vi "Cycle History Read.vi"(0 "GEA2 Reference In":refnum<k24>, 5 "Standalone?":bool, 6 "Cycle History Buffer Selection":T1, 11 "Error In":errorcluster) -> (4 "GEA2 Reference Out":refnum<k24>, 8 "output cluster":T2, 15 "Error Out":errorcluster)   [LabVIEW 2016, in "TL27.lvlib"]
uses:
  Projects/TL27.lvlib
  Q:/Common/DLLs/GEA3/GeaCommunication.dll
  Common/DLLs/GEA3/GeaCommunication.dll
  type defs/Cycle_Diag_Teststand.ctl
  type defs/Cycle History Buffer Selector.ctl
  Common/LabVIEW GEA2 Toolkit/LabVIEW_GEA2_Toolkit.lvlibp/type defs/Source_Destination.ctl
  Common/LabVIEW GEA2 Toolkit/LabVIEW_GEA2_Toolkit.lvlibp/type defs/ERD Read Data In.ctl
  Common/LabVIEW GEA2 Toolkit/LabVIEW_GEA2_Toolkit.lvlibp/type defs/Data Type.ctl
  Common/LabVIEW GEA2 Toolkit/LabVIEW_GEA2_Toolkit.lvlibp
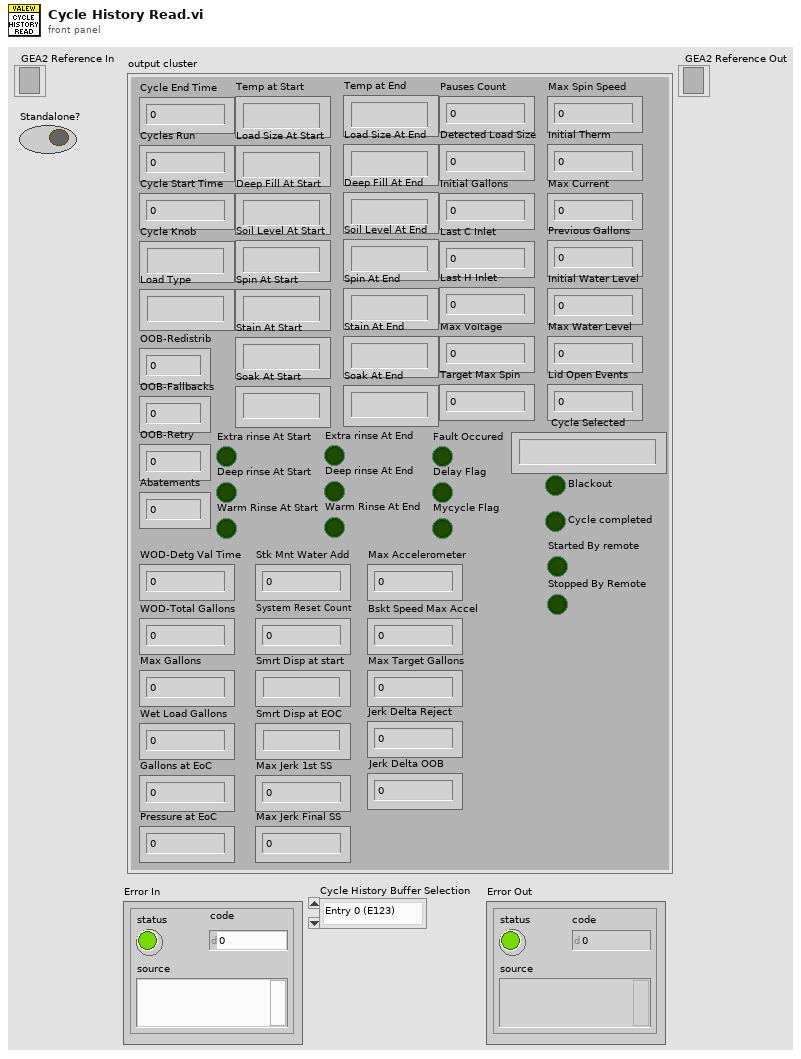
[diagram p1: front panel]
types:
  T1 = typedef "TL27.lvlib/Cycle History Buffer Selector.ctl" = enum16{"Entry 0 (E123)", "Entry 1 (E124)", "Entry 2 (E125)", "Entry 3 (E126)", "Entry 4 (E127)", "Entry 5 (E128)", "Entry 6 (E129)", "Entry 7 (E12A)", "Entry 8 (E12B)", "Entry 9 (E12C)"}
  T2 = typedef "TL27.lvlib/Cycle_Diag_Teststand.ctl" = cluster{"Cycle End Time":u32, "Cycles Run":u32, "Cycle Start Time":u32, "Cycle Knob":string, "Load Type":string, "OOB-Redistrib":u8, "OOB-Fallbacks":u8, "OOB-Retry":u8, "Temp at Start":string, "Load Size At Start":string, "Deep Fill At Start":string, "Soil Level At Start":string, "Spin At Start":string, "Extra rinse At Start":bool, "Deep rinse At Start":bool, "Stain At Start":string, "Soak At Start":string, "Warm Rinse At Start":bool, "Temp at End":string, "Load Size At End":string, "Deep Fill At End":string, "Soil Level At End":string, "Spin At End":string, "Extra rinse At End":bool, "Deep rinse At End":bool, "Stain At End":string, "Soak At End":string, "Warm Rinse At End":bool, "Pauses Count":u8, "Fault Occured":bool, "Delay Flag":bool, "Mycycle Flag":bool, "Blackout":bool, "Cycle completed":bool, "Detected Load Size":dbl, "Initial Gallons":dbl, "Last C Inlet ":dbl, "Max Voltage":dbl, "Target Max Spin":u16, "Max Spin Speed":u16, "Initial Therm":dbl, "Max Current":dbl, "Previous Gallons":dbl, "Initial Water Level":dbl, "Max Water Level":dbl, "Abatements ":u8, "Lid Open Events":u8, "Cycle Selected":string, "Last H Inlet ":dbl, "WOD-Detg Val Time":u8, "WOD-Total Gallons":u16, "Max Gallons":u16, "Wet Load Gallons":u16, "Gallons at EoC":u16, "Pressure at EoC":u32, "Stk Mnt Water Add":u8, "Started By remote":bool, "Stopped By Remote":bool, "System Reset Count":u8, "Smrt Disp at start":string, "Smrt Disp at EOC":string, "Max Jerk 1st SS":i32, "Max Jerk Final SS":i32, "Max Accelerometer":i16, "Bskt Speed Max Accel":u16, "Max Target Gallons":u16, "Jerk Delta Reject":u8, "Jerk Delta OOB ":u8}
  T3 = typedef "LabVIEW_GEA2_Toolkit.lvlibp/Source_Destination.ctl" = cluster{"Source":u8, "Destination":u8}
  T4 = typedef "LabVIEW_GEA2_Toolkit.lvlibp/ERD Read Data In.ctl" = cluster{"ERD Number":u16, "Data Type":T5}
  T5 = typedef "LabVIEW_GEA2_Toolkit.lvlibp/Data Type.ctl" = enum16{"string", "boolean", "uint8_t", "uint16_t", "uint32_t", "uint64_t", "int8_t", "int16_t", "int32_t", "int64_t"}
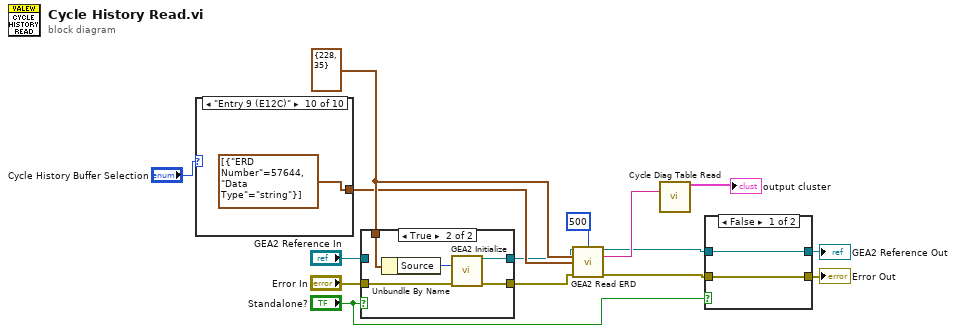
[diagram p0: block diagram]
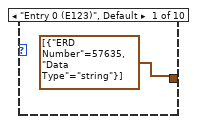
[diagram p2: hidden frame]
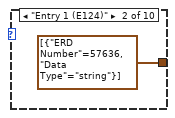
[diagram p3: hidden frame]
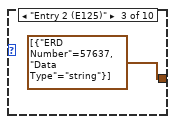
[diagram p4: hidden frame]
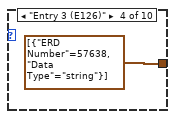
[diagram p5: hidden frame]
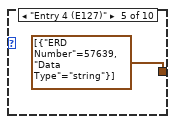
[diagram p6: hidden frame]
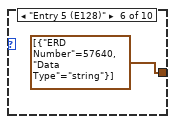
[diagram p7: hidden frame]
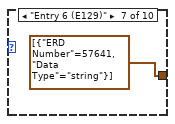
[diagram p8: hidden frame]
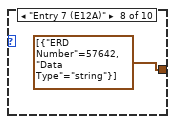
[diagram p9: hidden frame]
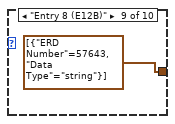
[diagram p10: hidden frame]
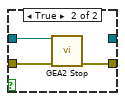
[diagram p11: hidden frame]
diagram:
  w9 = T3 {"Source"=228, "Destination"=35} ("GEA Inputs")
  n1 = case shown="\"Entry 9 (E12C)\"" "Cycle History Buffer Selection" {
    tunnel: [T4[] [{"ERD Number"=57635, "Data Type"=enum."string"}] ("Read ERD List") T4[] [{"ERD Number"=57636, "Data Type"=enum."string"}] ("Read ERD List") T4[] [{"ERD Number"=57637, "Data Type"=enum."string"}] ("Read ERD List") T4[] [{"ERD Number"=57638, "Data Type"=enum."string"}] ("Read ERD List") T4[] [{"ERD Number"=57639, "Data Type"=enum."string"}] ("Read ERD List") T4[] [{"ERD Number"=57640, "Data Type"=enum."string"}] ("Read ERD List") T4[] [{"ERD Number"=57641, "Data Type"=enum."string"}] ("Read ERD List") T4[] [{"ERD Number"=57642, "Data Type"=enum."string"}] ("Read ERD List") T4[] [{"ERD Number"=57643, "Data Type"=enum."string"}] ("Read ERD List") T4[] [{"ERD Number"=57644, "Data Type"=enum."string"}] ("Read ERD List")] -> w7
    frame "Entry 0 (E123)", Default {
    }
    frame "Entry 1 (E124)" {
    }
    frame "Entry 2 (E125)" {
    }
    frame "Entry 3 (E126)" {
    }
    frame "Entry 4 (E127)" {
    }
    frame "Entry 5 (E128)" {
    }
    frame "Entry 6 (E129)" {
    }
    frame "Entry 7 (E12A)" {
    }
    frame "Entry 8 (E12B)" {
    }
    frame "Entry 9 (E12C)" {
    }
  }
  n2 = case shown="True" "Standalone?" {
    tunnel: "Error In" -> [w26 w32]
    tunnel: [w26 w31] -> w10
    tunnel: "GEA2 Reference In" -> [w27 _]
    tunnel: [w27 w30] -> w6
    tunnel: w9 -> [_ w28]
    frame False {
    }
    frame True {
      n3 = Unbundle By Name(w28) -> ("Source"=w29:u8)
      n4 = call "GEA2 Initialize.vi"("Source Address"=w29, "error in"=w32) -> ("GEA2 Reference Out"=w30:refnum<k24>, "error out"=w31:errorcluster)  [unwired: 11 in, 1 out]
    }
  }
  n5 = call "GEA2 Read ERD.vi"("GEA2 Reference In"=w6, "Read Timeout (ms)"=u32 500, "GEA Inputs"=w9, "Read ERD List"=w7, "Error In"=w10) -> ("GEA2 Reference Out"=w4:refnum<k24>, "Raw Data Out"=w5:string, "Error Out"=w3:errorcluster)  [unwired: 7 in, 1 out]
  n6 = call "Cycle Diag Table Read.vi"("Raw Data In"=w5) -> ("output cluster"=→"output cluster":T2)  [unwired: 14 in]
  n7 = case shown="False" "Standalone?" {
    tunnel: [w33 w37] -> w13
    tunnel: w4 -> [w34 w36]
    tunnel: [w34 _] -> w12
    tunnel: w3 -> [w33 w35]
    frame False {
    }
    frame True {
      n8 = call "GEA2 Stop.vi"("GEA2 Reference In"=w36, "Error In"=w35) -> ("Error Out"=w37:errorcluster)  [unwired: 13 in]
    }
  }
  "Error Out" <- w13
  "GEA2 Reference Out" <- w12
